vi "Render Picture.vi"(11 "Point in":refnum<class "Point.lvclass">) -> (1 "Picture":picture, 3 "Point out":refnum<class "Point.lvclass">)   [LabVIEW 2018, in "Point.lvclass"]
doc: "Render the point into the picture."
uses:
  Point.lvclass
  Point.lvclass/Point.ctl
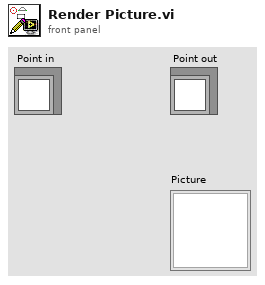
[diagram p1: front panel]
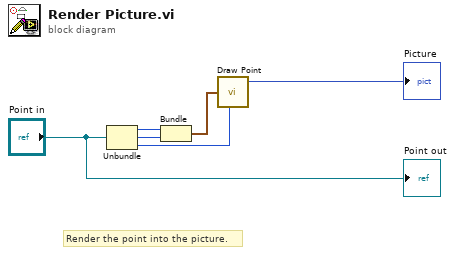
[diagram p0: block diagram]
diagram:
  # "Render the point into the picture."
  n1 = Unbundle("Point in") -> (w4:i16, w3:i16, w2:u32)
  n2 = Bundle("X"=w4, "Y"=w3) -> (w5:cluster{"X":i16, "Y":i16})  [unwired: 1 out]
  n3 = call <vilib>:"Draw Point.vi"("point(x,y)"=w5, "color(black)"=w2) -> ("new picture"=→"Picture":picture)  [unwired: 2 in, 5 out]
  "Point out" <- "Point in"
